vi "AlliGator Optimal IRF Metrics.vi"(8 "Error In":errorcluster, 9 "index":i32, 10 "Smooth Metrics":bool, 11 "Plot Array":cluster{"X Array":dbl[], "Y Array":dbl[]}[](array[cluster])) -> (0 "Error Out":errorcluster, 2 "Message":string)   [LabVIEW 2021, in "AlliGator IRF.lvlib"]
uses:
  AlliGator IRF.lvlib
  AlliGator IRF Deconvolution Metrics.ctl
panel:
  in  "Metrics":T1
  # "see the License on the block diagram (Ctrl+E or Window:Show Block Diagram)"
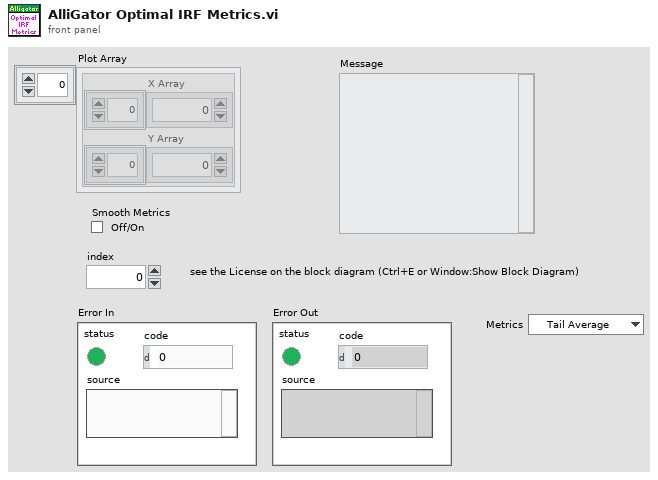
[diagram p1: front panel]
types:
  T1 = typedef "AlliGator IRF.lvlib/AlliGator IRF Deconvolution Metrics.ctl" = enum16{"Tail Average", "Tail SDV", "Tail Max", "Tail Average * SDV", "Tail Slope", "Residuals ACF SDV", "Delta tau", "Reduced Chi2", "Residuals Area"}
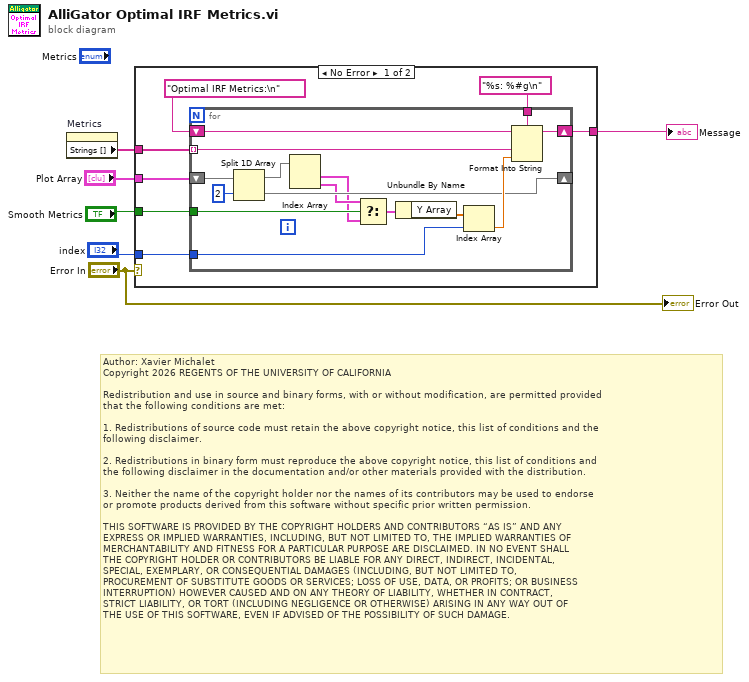
[diagram p0: block diagram]
diagram:
  # "Author: Xavier Michalet\nCopyright 2026 REGENTS OF THE UNIVERSITY OF CALIFORNIA\n\nRedistribution and use in source and binary forms, with or without modification, are permitted provided\nthat the following conditions are met:\n\n1. Redistributions of source code must retain the above copyright notice, this list of conditions and the\nfollowing disclaimer.\n\n2. Redistributions in binary form must reproduce the above copyright notice, this list of conditions and\nthe following disclaimer in the documentation and/or other materials provided with the distribution.\n\n3. Neither the name of the copyright holder nor the names of its contributors may be used to endorse \nor promote products derived from this software without specific prior written permission.\n\nTHIS SOFTWARE IS PROVIDED BY THE COPYRIGHT HOLDERS AND CONTRIBUTORS “AS IS” AND ANY \nEXPRESS OR IMPLIED WARRANTIES, INCLUDING, BUT NOT LIMITED TO, THE IMPLIED WARRANTIES OF\nMERCHANTABILITY AND FITNESS FOR A PARTICULAR PURPOSE ARE DISCLAIMED. IN NO EVENT SHALL\nTHE COPYRIGHT HOLDER OR CONTRIBUTORS BE LIABLE FOR ANY DIRECT, INDIRECT, INCIDENTAL, \nSPECIAL, EXEMPLARY, OR CONSEQUENTIAL DAMAGES (INCLUDING, BUT NOT LIMITED TO, \nPROCUREMENT OF SUBSTITUTE GOODS OR SERVICES; LOSS OF USE, DATA, OR PROFITS; OR BUSINESS\nINTERRUPTION) HOWEVER CAUSED AND ON ANY THEORY OF LIABILITY, WHETHER IN CONTRACT, \nSTRICT LIABILITY, OR TORT (INCLUDING NEGLIGENCE OR OTHERWISE) ARISING IN ANY WAY OUT OF\nTHE USE OF THIS SOFTWARE, EVEN IF ADVISED OF THE POSSIBILITY OF SUCH DAMAGE."
  n1 = property on="Metrics" class="Enum (strict)"() -> ("Strings []"=w6:string[])  [unwired: 2 in, 2 out]
  n2 = case shown="No Error" "Error In" {
    tunnel: w6 -> [w13 _]
    tunnel: "Plot Array" -> [w11 _]
    tunnel: "index" -> [w10 _]
    tunnel: "Smooth Metrics" -> [w9 _]
    tunnel: [w8 _] -> w2
    frame No Error {
      n3 = for {
        tunnel: w13 -> [w28] mode=indexing
        tunnel: "%s: %#g\n" ("format string") -> [w27]
        tunnel: w10 -> [w25]
        shift-right: [w21] -> _
        shift-left: w11 -> [w23]
        tunnel: w9 -> [w19]
        shift-right: [w15] -> w8
        shift-left: "Optimal IRF Metrics:\n" ("format string") -> [w14]
        n4 = Split 1D Array(array=w23, index=2) -> (first subarray=w20:cluster{"X Array":dbl[], "Y Array":dbl[]}[], second subarray=w21:cluster{"X Array":dbl[], "Y Array":dbl[]}[])
        n5 = Index Array(array=w20) -> (element #1=w17:cluster{"X Array":dbl[], "Y Array":dbl[]}, element #2=w18:cluster{"X Array":dbl[], "Y Array":dbl[]})  [unwired: 2 in]
        n6 = Select(t=w18, s=w19, f=w17) -> (s? t:f=w16:cluster{"X Array":dbl[], "Y Array":dbl[]})
        n7 = Unbundle By Name(w16) -> ("Y Array"=w26:dbl[])
        n8 = Index Array(array=w26, index=w25) -> (element=w24:dbl)
        n9 = Format Into String(format string=w27, initial string=w14, w28, w24) -> (resulting string=w15:string)  [unwired: 1 in, 1 out]
      }
    }
    frame Error {
    }
  }
  "Message" <- w2
  "Error Out" <- "Error In"
